vi "idn_action.vi"(0 "HGF_ImaqFg":refnum<class "HGF_ImaqFg.lvclass">, 5 "error in (no error)":errorcluster) -> (12 "resourceString":string, 13 "additionalInfo":string, 14 "HGF_ImaqFg out":refnum<class "HGF_ImaqFg.lvclass">, 15 "driverRevision":string="unknown", 16 "firmwareRevision":string="unknown", 17 "vendor":string="unknown", 18 "model":string="unknown", 19 "error out":errorcluster)   [LabVIEW 2014, in "HGF_IMAQ.lvlib" / "HGF_ImaqFg.lvclass"]
doc: "This VI queries the current instrument firmware revision and instrument driver revision.\n\nFor detailed driver information including modification history, refer to the Readme file.\n\n<b>Hint:</b> This is a dynamic dispatch VI to be implemented by child classes."
uses:
  HGF_ImaqFg.lvclass
  HGF_IMAQDevice/HGF_IMAQDevice.lvclass
panel:
  in  "Interface Type":i32(ring)=5125 items=["1405"=5125, "1407"=5127, "1408"=5128, "1409"=5129, "1410"=5136, "1411"=5137, "1422"=5154, "1424"=5156, "1426"=5158, "1427"=5159, "1428"=5160, "1429"=5161, "1430"=5168, "1722"=5922, "1742"=5954, "1762"=5986]
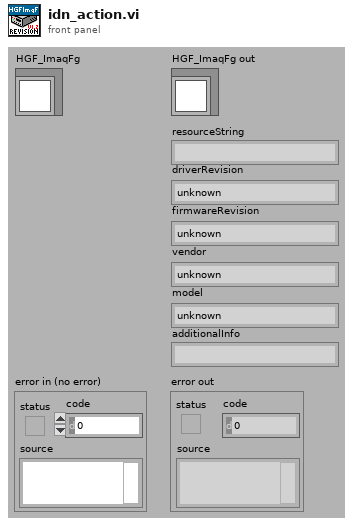
[diagram p1: front panel]
types:
  T1 = cluster{"Major":u16, "Minor":u16, "Fix":u16, "Build":u16}
  T2 = typedef "LVStringsAndValuesArrayTypeDef_I32.ctl" = cluster{"String":string, "Value":i32}[]
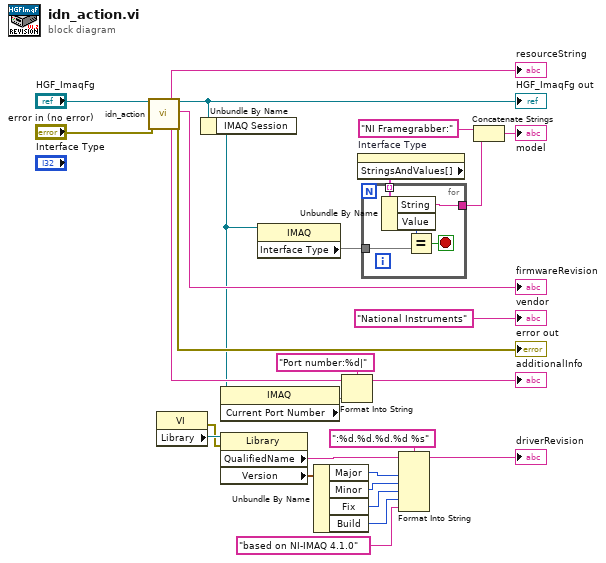
[diagram p0: block diagram]
diagram:
  n1 = call-parent "idn_action.vi"("HGF_IMAQDevice"="HGF_ImaqFg", "error in (no error)"="error in (no error)") -> ("resourceString"=→"resourceString":string, "additionalInfo"=w25:string, "HGF_IMAQDevice out"=w22:refnum<class "HGF_ImaqFg.lvclass">, "firmwareRevision"=→"firmwareRevision":string, "error out"=→"error out":errorcluster)  [unwired: 13 out]
  "HGF_ImaqFg out" <- w22
  n2 = property class="VI"() -> (error out=w10:errorcluster, "Library"=w14:refnum<vi>)  [unwired: 2 in, 1 out]
  n3 = Unbundle By Name(w22) -> ("IMAQ Session"=w5:refnum<k11>)
  n4 = property class="IMAQ"(reference=w5) -> ("Current Port Number"=w8)  [unwired: 1 in, 2 out]
  n5 = property class="Library"(reference=w14, error in=w10) -> ("QualifiedName"=w12:string, "Version"=w20:T1)  [unwired: 2 out]
  n6 = property class="IMAQ"(reference=w5) -> ("Interface Type"=w4)  [unwired: 1 in, 2 out]
  n7 = Unbundle By Name(w20) -> ("Major"=w19:u16, "Minor"=w18:u16, "Fix"=w17:u16, "Build"=w16:u16)
  n8 = Format Into String(format string="Port number:%d|", initial string=w25, w8) -> (resulting string=→"additionalInfo":string)  [unwired: 1 in, 1 out]
  n9 = property on="Interface Type" class="Ring (strict)"() -> ("StringsAndValues[]"=w6:T2)  [unwired: 2 in, 2 out]
  n10 = for {
    tunnel: w6 -> [w33] mode=indexing
    tunnel: w4 -> [w31]
    tunnel: [w29] -> w2
    stop <- w30 stop-if-true
    n11 = Unbundle By Name(w33) -> ("String"=w29:string, "Value"=w32:i32)
    n12 = Equal?(x=w32, y=w31) -> (x = y?=w30:bool)
  }
  n13 = Format Into String(format string=":%d.%d.%d.%d %s", initial string=w12, w19, w18, w17, w16, "based on NI-IMAQ 4.1.0" ("driverRevision")) -> (resulting string=→"driverRevision":string)  [unwired: 1 in, 1 out]
  n14 = Concatenate Strings("NI Framegrabber:" ("model"), w2) -> (→"model":string)
  "vendor" <- "National Instruments" ("vendor")
